vi "Option selector and writer in Stdby.vi"(0 ".NET Refnum in":refnum<k24>, 5 "Option Selection":T1, 7 "ECT Parameters":T2={"MS to Spin Time"=0, "Target Fill Time"=0, "MS to Agitate Time"=0, "MS to Spin before Spin Time "=0, "Adaptive Drain Time"=60, "Coast to 0 Time"=60}, 11 "error in (no error)":errorcluster) -> (4 ".NET Refnum out":refnum<k24>, 6 "ECT Pass/Fail":bool, 8 "Report Text":string, 12 "Actual ECT (sec)":u16, 13 "Expected ECT (sec)":u16, 14 "Expected SSD":string, 15 "error out":errorcluster)   [LabVIEW 2016, in "TLMB.lvlib"]
uses:
  Projects/TLMB.lvlib
  Q:/Common/DLLs/GEA3/GeaCommunication.dll
  Common/DLLs/GEA3/GeaCommunication.dll
  Controls/ECT Parameters.ctl
  Controls/Options.ctl
  Common/LabVIEW GEA2 Toolkit/LabVIEW_GEA2_Toolkit.lvlibp/type defs/ERD Read Data In.ctl
  Common/LabVIEW GEA2 Toolkit/LabVIEW_GEA2_Toolkit.lvlibp/type defs/Data Type.ctl
  Common/LabVIEW GEA2 Toolkit/LabVIEW_GEA2_Toolkit.lvlibp/type defs/Source_Destination.ctl
  Common/LabVIEW GEA2 Toolkit/LabVIEW_GEA2_Toolkit.lvlibp
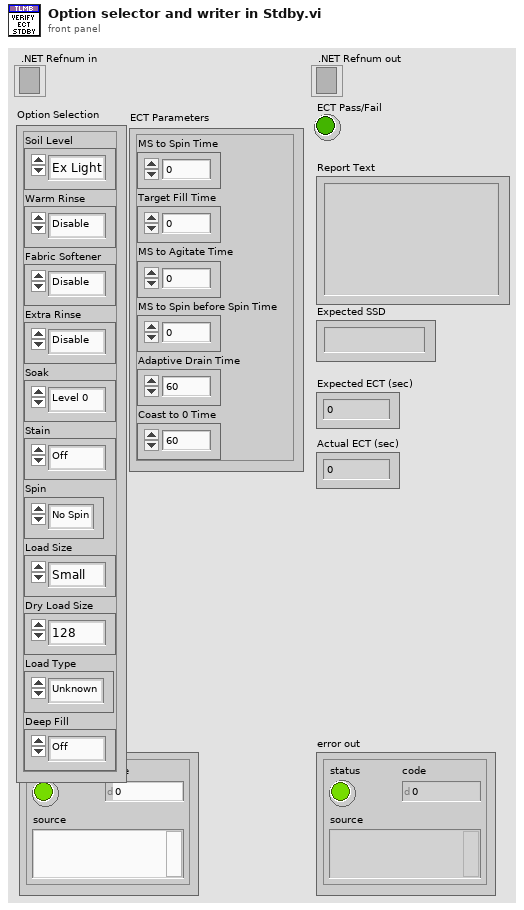
[diagram p1: front panel]
types:
  T1 = typedef "TLMB.lvlib/Options.ctl" = cluster{"Soil Level":enum8{"Ex Light", "Light", "Normal", "Heavy", "Ex Heavy"}, "Warm Rinse":enum8{"Disable", "Enable"}, "Fabric Softener":enum16{"Disable", "Enable"}, "Extra Rinse":enum8{"Disable", "Enable"}, "Soak":enum8{"Level 0", "Level 1", "Level 2", "Level 3", "Level 4"}, "Stain":enum8{"Off", "Tomato", "Wine", "Blood", "Grass", "Dirt"}, "Spin":enum16{"No Spin", "Normal Spin", "More Spin", "Max Spin"}, "Load Size":enum8{"Small", "Medium", "Large", "Super", "Precise Fill", "Super Plus"}, "Dry Load Size":enum16{"128", "256", "384", "5AA", "6A4", "834", "65535"}, "Load Type":enum8{"Unknown", "Cotton", "Synthetic", "Mixed", "Wet", "Low Flow", "Small", "Medium", "Large", "Super", "Super Plus", "Max"}, "Deep Fill":enum8{"Off", "Incremental Fill", "Max Fill"}}
  T2 = typedef "TLMB.lvlib/ECT Parameters.ctl" = cluster{"MS to Spin Time":u16, "Target Fill Time":u16, "MS to Agitate Time":u16, "MS to Spin before Spin Time ":u16, "Adaptive Drain Time":u16, "Coast to 0 Time":u16}
  T3 = typedef "LabVIEW_GEA2_Toolkit.lvlibp/Source_Destination.ctl" = cluster{"Source":u8, "Destination":u8}
  T4 = typedef "LabVIEW_GEA2_Toolkit.lvlibp/ERD Read Data In.ctl" = cluster{"ERD Number":u16, "Data Type":T5}
  T5 = typedef "LabVIEW_GEA2_Toolkit.lvlibp/Data Type.ctl" = enum16{"string", "boolean", "uint8_t", "uint16_t", "uint32_t", "uint64_t", "int8_t", "int16_t", "int32_t", "int64_t"}
  T6 = typedef "LabVIEW_GEA2_Toolkit.lvlibp/ERD Write Data In.ctl" = cluster{"ERD Number":u16, "Data Type":T5, "Data":string}
  T7 = typedef "TLMB.lvlib/ECT.ctl" = cluster{"MS to Agitate Time":u16, "Adaptive Drain Time":u16, "Coast to 0 Time":u16, "Agitate Time":u16, "Warm Rinse Time":u16, "FS Time":u16, "Ex Rinse Time":u16, "Soak Time":u16, "Stain Time":u16, "Motor Profile ID":u16, "Calculated ECT":u16, "Spin Time":u16}
  T8 = typedef "LabVIEW_GEA2_Toolkit.lvlibp/ERD Read Data Out.ctl" = cluster{"ERD Number":u16, "Data":string}
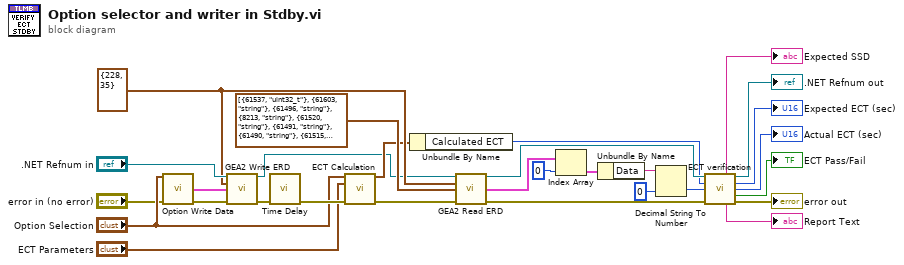
[diagram p0: block diagram]
diagram:
  w8 = T3 {"Source"=228, "Destination"=35} ("GEA Inputs")
  n1 = call "Option Write Data.vi"("Option Selection"="Option Selection", "Error In"="error in (no error)") -> ("appended array"=w11:T6[], "Error Out"=w3:errorcluster)  [unwired: 12 in]
  n2 = call "GEA2 Write ERD.vi"("GEA2 Reference In"=".NET Refnum in", "GEA Inputs"=w8, "Write ERD List"=w11, "Error In"=w3) -> ("GEA2 Reference Out"=w6:refnum<k24>, "Error Out"=w9:errorcluster)  [unwired: 9 in, 1 out]
  n3 = call "Time Delay"("error in (no error)"=w9) -> ("error out"=w12:errorcluster)  [unwired: 10 in]
  n4 = call "ECT Calculation.vi"("Option Selection"="Option Selection", "ECT Parameters"="ECT Parameters", "Error In"=w12) -> ("Expected ECT"=w7:T7, "Error Out"=w26:errorcluster)  [unwired: 11 in]
  n5 = Unbundle By Name(w7) -> ("Calculated ECT"=w19:u16)
  n6 = call "GEA2 Read ERD.vi"("GEA2 Reference In"=w6, "GEA Inputs"=w8, "Read ERD List"=T4[] [{"ERD Number"=61537, "Data Type"=enum."uint32_t"}, {"ERD Number"=61603, "Data Type"=enum."string"}, {"ERD Number"=61496, "Data Type"=enum."string"}, {"ERD Number"=8213, "Data Type"=enum."string"}, {"ERD Number"=61520, "Data Type"=enum."string"}, {"ERD Number"=61491, "Data Type"=enum."string"}, {"ERD Number"=61490, "Data Type"=enum."string"}, {"ERD Number"=61515, "Data Type"=enum."string"}, {"ERD Number"=61494, "Data Type"=enum."string"}, {"ERD Number"=61493, "Data Type"=enum."string"}], "Error In"=w26) -> ("GEA2 Reference Out"=w25:refnum<k24>, "ERD Data Out"=w14:T8[], "Error Out"=w27:errorcluster)  [unwired: 8 in, 1 out]
  n7 = Index Array(array=w14, index=0) -> (element=w16:T8)
  n8 = Unbundle By Name(w16) -> ("Data"=w17:string)
  n9 = Decimal String To Number(string=w17, default (0L)=u16 0 ("default (0 I32)")) -> (number=w18:u16)  [unwired: 1 in, 1 out]
  n10 = call "ECT verification.vi"(".NET Refnum in"=w25, "Cal ECT (sec)"=w19, "Time remaining (sec)"=w18, "error in"=w27) -> ("Expected SSD"=→"Expected SSD":string, ".NET Refnum out"=→".NET Refnum out":refnum<k24>, "Expected ECT (sec)"=→"Expected ECT (sec)":u16, "Actual ECT (sec)"=→"Actual ECT (sec)":u16, "ECT Pass/Fail"=→"ECT Pass/Fail":bool, "Report Text"=→"Report Text":string, "error out"=→"error out":errorcluster)  [unwired: 5 in]
